vi "5492_ZeroYaw.vi"(8 "error in (no error)":errorcluster) -> (0 "error out":errorcluster)   [LabVIEW 2016]
uses:
  5492_InitialYaw.vi
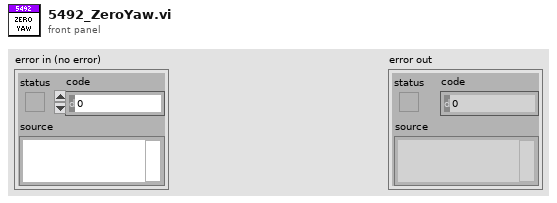
[diagram p1: front panel]
types:
  T1 = cluster{"Yaw":dbl, "Roll":dbl, "Pitch":dbl, "Heading":dbl, "Fused Heading":dbl}
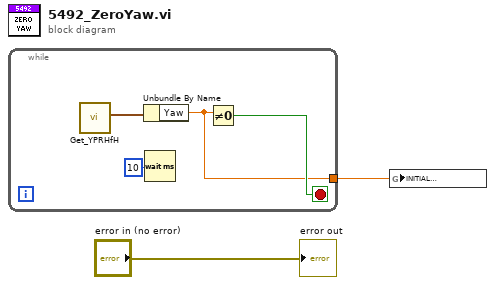
[diagram p0: block diagram]
diagram:
  n1 = while {
    tunnel: [w4] -> w2
    stop <- w5 stop-if-true
    n2 = call <vilib>:"Get_YPRHfH.vi"() -> ("YRPHfH"=w6:T1)  [unwired: 11 in]
    n3 = Unbundle By Name(w6) -> ("Yaw"=w4:dbl)
    n4 = Wait (ms)(milliseconds to wait=10) -> ()  [unwired: 1 out]
    n5 = Not Equal To 0?(x=w4) -> (x != 0?=w5:bool)
  }
  n6 = global write "5492_InitialYaw.vi" "INITIAL\n YAW"(w2) -> ()
  "error out" <- "error in (no error)"
